vi "Steinhart-Hart.vi"(8 "error in":errorcluster, 10 "Tref (C)":dbl[](array[numeric])=[50.0, 25.0, 0.0], 11 "R (kO)":dbl[](array[numeric])=[3.893, 10.0, 29.49]) -> (0 "error out":errorcluster, 3 "Coefficients":dbl[](array[numeric])=[0.0027277775126833296, 0.00026869922732867234, 6.173036108113934e-07] format="%.10e")   [LabVIEW 2018, in "Temperature.lvlib"]
doc: "Solves the Steinhart-Hart equation for the coefficients which determine the temperature coming off of the therimstor as a function of measured resistance."
uses:
  Temperature.lvlib
  <vilib>/Analysis/baseanly.llb/Matrix Type of Inverse Matrix.ctl
  <vilib>/Analysis/7linalg.llb/Solve Linear Equations (single right hand).vi
  <vilib>/Analysis/baseanly.llb/Solve Linear Equations By Cholesky.vi
  <vilib>/Analysis/baseanly.llb/Real Matrix to Compact Array.vi
  <vilib>/Analysis/baseanly.llb/Real Compact Tri-Matrix Linear Eqs.vi
  <vilib>/Analysis/Matrix/Numeric/Conversions/Array To Matrix - RA2.vi
  <vilib>/Analysis/7linalg.llb/Solve Linear Eqs (General).vi
  <vilib>/Analysis/7linalg.llb/Solve Linear Eqs (Gen, single right hand).vi
  <vilib>/Analysis/NI_AALPro.lvlib
  <vilib>/Analysis/NI_AALBase.lvlib
  <vilib>/Analysis/Matrix/NI_Matrix.lvlib
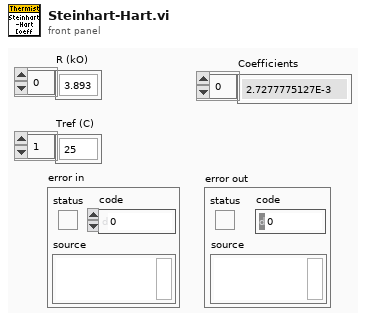
[diagram p1: front panel]
types:
  T1 = typedef "NI_AALBase.lvlib/Matrix Type of Inverse Matrix.ctl" = enum32{"General", "Positive Definite", "Lower Triangular", "Upper Triangular"}
  T2 = typedef "NI_Matrix.lvlib/RealMatrix.ctl" = dbl[][]
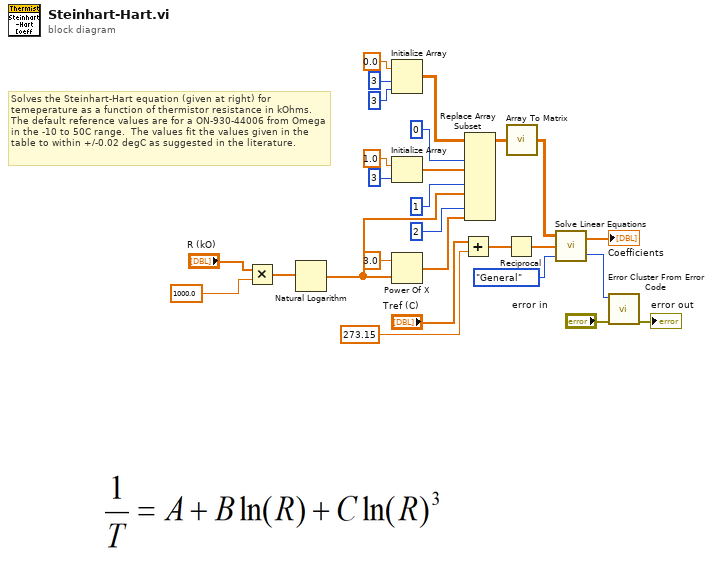
[diagram p0: block diagram]
diagram:
  # "Solves the Steinhart-Hart equation (given at right) for temeperature as a function of thermistor resistance in kOhms.  The default reference values are for a ON-930-44006 from Omega in the -10 to 50C range.  The values fit the values given in the table to within +/-0.02 degC as suggested in the literature."
  n1 = Multiply(x="R (kO)", y=1000.0) -> (x*y=w2:dbl[])
  n2 = Natural Logarithm(1:w2) -> (0:w8:dbl[])
  n3 = Initialize Array(0.0 ("element"), 3 ("dimension size"), 3 ("dimension size")) -> (w20:dbl[][])
  n4 = Initialize Array(1.0 ("element"), 3 ("dimension size")) -> (w17:dbl[])
  n5 = Power Of X(1:w8, 2:3.0) -> (0:w15:dbl[])
  n6 = Add(x="Tref (C)", y=273.15) -> (x+y=w7:dbl[])
  n7 = Replace Array Subset(array=w20, new element #1=w17, index (col) #1=0 ("disabled index (col)"), new element #2=w8, index (col) #2=1 ("index (col)"), new element #3=w15, index (col) #3=2 ("index (col)")) -> (w14:dbl[][])  [unwired: 3 in]
  n8 = Reciprocal(x=w7) -> (1/x=w25:dbl[])
  n9 = call-poly <vilib>:"Array To Matrix.vi"("Real 2D Array"=w14) -> ("Real Matrix"=w13:T2)
  n10 = call-poly <vilib>:"Solve Linear Equations.vi"("matrix type"=Matrix_Type_of_Inverse_Matrix."General", "Known Vector"=w25, "Input Matrix"=w13) -> ("error"=w12:i32, "Solution Vector"=→"Coefficients":dbl[])
  n11 = call <vilib>:"Error Cluster From Error Code.vi"("error in (no error)"="error in", "error code (0)"=w12) -> ("error out"=→"error out":errorcluster)  [unwired: 1 in, 6 out]
